vi "Cascade To Direct Coefficients.vi"(0 "IIR Filter Cluster":T1 {"Forward Coefficients" format="%.4f"; "Reverse Coefficients" format="%.4f"}) -> (1 "Reverse Coefficients":dbl[](array[numeric]), 2 "Forward Coefficients":dbl[](array[numeric]))   [LabVIEW 2020, in "NI_AALBase.lvlib"]
doc: "Converts IIR filter coefficients from the cascade form to the direct form."
uses:
  <vilib>/Analysis/NI_AALBase.lvlib
  <vilib>/Analysis/2dsp.llb/1D Convolution (DBL).vi
  <vilib>/Analysis/NI_AALPro.lvlib
panel:
  # "Cascade->Direct Coefficients"
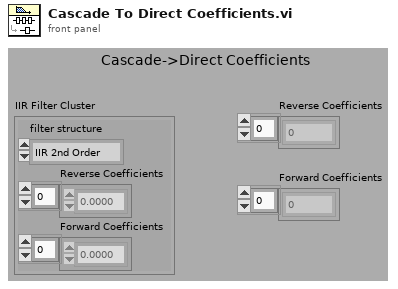
[diagram p1: front panel]
types:
  T1 = cluster{"filter structure":enum32{"IIR 2nd Order", "IIR 4th Order"}, "Reverse Coefficients":dbl[], "Forward Coefficients":dbl[]}
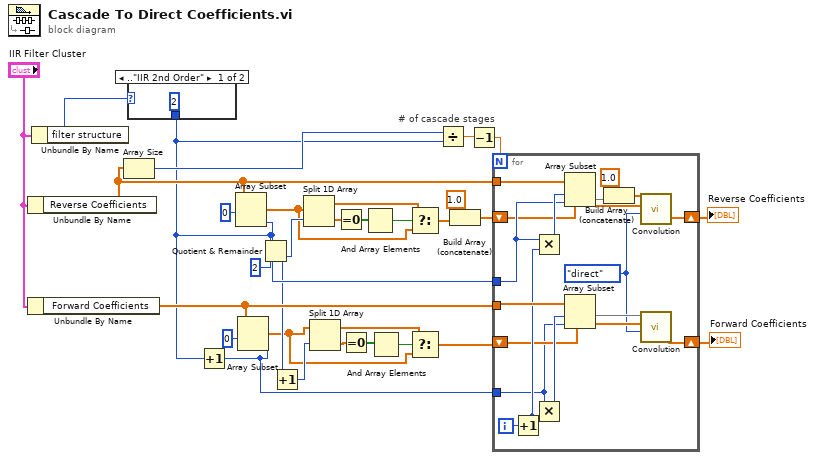
[diagram p0: block diagram]
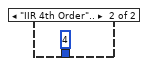
[diagram p2: hidden frame]
diagram:
  # "# of cascade stages"
  n1 = Unbundle By Name("IIR Filter Cluster") -> ("Reverse Coefficients"=w18:dbl[])
  n2 = Unbundle By Name("IIR Filter Cluster") -> ("Forward Coefficients"=w22:dbl[])
  n3 = Unbundle By Name("IIR Filter Cluster") -> ("filter structure"=w30:enum32{"IIR 2nd Order", "IIR 4th Order"})
  n4 = Array Size(array=w18) -> (size(s)=w29:i32)
  n5 = case shown="..\"IIR 2nd Order\"" w30 {
    tunnel: [2 4] -> w11
    frame .."IIR 2nd Order" {
    }
    frame "IIR 4th Order".. {
    }
  }
  n6 = Increment(x=w11) -> (x+1=w2:i32)
  n7 = Array Subset(array=w18, index=0, length=w11) -> (w6:dbl[])
  n8 = Array Subset(array=w22, index=0, length=w2) -> (w4:dbl[])
  n9 = Quotient & Remainder(x=w11, y=2) -> (floor(x/y)=w9:i32)  [unwired: 1 out]
  n10 = Increment(x=w9) -> (x+1=w10:i32)
  n11 = Split 1D Array(array=w6, index=w9) -> (first subarray=w7:dbl[], second subarray=w17:dbl[])
  n12 = Split 1D Array(array=w4, index=w10) -> (first subarray=w5:dbl[], second subarray=w13:dbl[])
  n13 = Equal To 0?(x=w17) -> (x = 0?=w16:bool[])
  n14 = Equal To 0?(x=w13) -> (x = 0?=w14:bool[])
  n15 = And Array Elements(Boolean array=w16) -> (logical AND=w15:bool)
  n16 = And Array Elements(Boolean array=w14) -> (logical AND=w8:bool)
  n17 = Select(t=w7, s=w15, f=w6) -> (s? t:f=w19:dbl[])
  n18 = Select(t=w5, s=w8, f=w4) -> (s? t:f=w3:dbl[])
  n19 = Divide(x=w29, y=w11) -> (x/y=w28:dbl)
  n20 = Build Array (concatenate)(1.0, w19) -> (w20:dbl[])
  n21 = Decrement(x=w28) -> (x-1=w27:dbl)
  n22 = for {
    N: w27 -> [_]
    shift-right: [w41] -> w24
    shift-left: w20 -> [w42]
    tunnel: w11 -> [w45]
    tunnel: w18 -> [w44]
    shift-right: [w40] -> w21
    shift-left: w3 -> [w36]
    tunnel: w22 -> [w39]
    tunnel: w2 -> [w34]
    i -> [w46]
    w33 = enum32{"direct", "frequency domain"}."direct" ("algorithm")
    n23 = Increment(x=w46) -> (x+1=w38:i32)
    n24 = Multiply(x=w45, y=w38) -> (x*y=w47:i32)
    n25 = Multiply(x=w34, y=w38) -> (x*y=w37:i32)
    n26 = Array Subset(array=w44, index=w47, length=w45) -> (w49:dbl[])
    n27 = Array Subset(array=w39, index=w37, length=w34) -> (w35:dbl[])
    n28 = Build Array (concatenate)(1.0, w49) -> (w43:dbl[])
    n29 = call-poly <vilib>:"Convolution.vi"("algorithm"=w33, "Y"=w42, "X"=w43) -> ("X * Y"=w41:dbl[])  [unwired: 7 in, 1 out]
    n30 = call-poly <vilib>:"Convolution.vi"("algorithm"=w33, "Y"=w36, "X"=w35) -> ("X * Y"=w40:dbl[])  [unwired: 7 in, 1 out]
  }
  "Reverse Coefficients" <- w24
  "Forward Coefficients" <- w21
